vi "Get Source Files And Folders.vi"(8 "Error In":errorcluster, 11 "Configuration":T1) -> (0 "Error Out":errorcluster, 1 "All Source Folders":path[](array[path]), 2 "All Source Files":path[](array[path]), 3 "Configuration":T1)   [LabVIEW 2011, in "LVH-Build-Tools.lvlib"]
uses:
  LVH-Build-Tools.lvlib
  Type Defs/Configuration.ctl
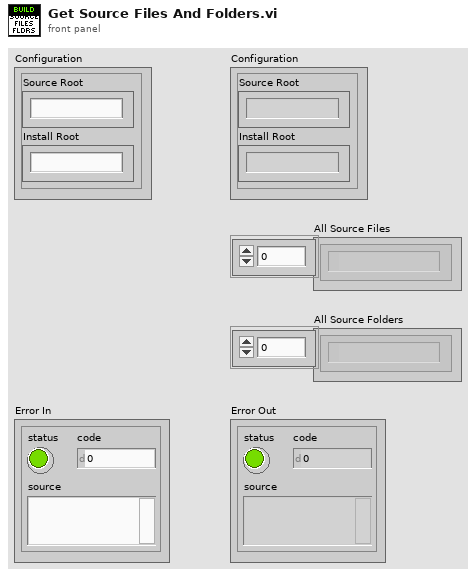
[diagram p1: front panel]
types:
  T1 = typedef "LVH-Build-Tools.lvlib/Configuration.ctl" = cluster{"Source Root":string, "Install Root":string, "Components":string[], "Ignore":string[]}
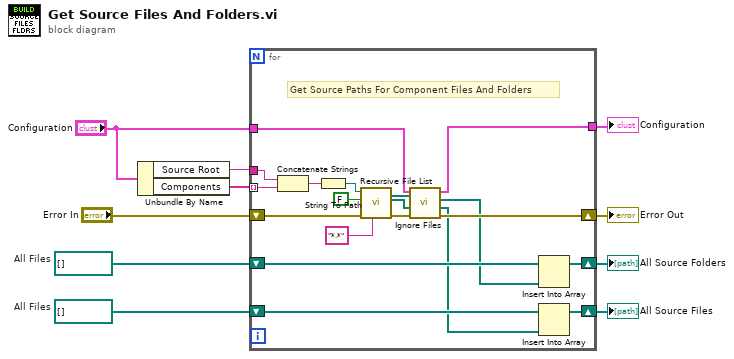
[diagram p0: block diagram]
diagram:
  w7 = path[] []  # All Files
  w6 = path[] []  # All Files
  n1 = Unbundle By Name("Configuration") -> ("Source Root"=w4:string, "Components"=w3:string[])
  n2 = for {
    tunnel: w3 -> [w17] mode=indexing
    tunnel: w4 -> [w18]
    shift-right: [w23] -> w8
    shift-left: w6 -> [w22]
    shift-right: [w20] -> w10
    shift-left: w7 -> [w21]
    shift-right: [w19] -> w9
    shift-left: "Error In" -> [w24]
    tunnel: "Configuration" -> [w14]
    tunnel: [w13] -> w1
    # "Get Source Paths For Component Files And Folders"
    n3 = Concatenate Strings(w18, w17) -> (w25:string)
    n4 = String To Path(string=w25) -> (path=w26:path)
    n5 = call <vilib>:"Recursive File List.vi"("pattern"="*.*", "error in (no error)"=w24, "Treat LLBs as Folders?"=FALSE, "Folder Path"=w26) -> ("error out"=w29:errorcluster, "All Files in Dir"=w15:path[], "All Folders"=w16:path[])  [unwired: 3 in, 2 out]
    n6 = call "Ignore Files.vi"("Error In"=w29, "All Files"=w15, "All Folders"=w16, "Configuration"=w14) -> ("Error Out"=w19:errorcluster, "All Files"=w11:path[], "All Folders"=w12:path[], "Configuration"=w13:T1)  [unwired: 4 in]
    n7 = Insert Into Array(array=w22, new element=w12) -> (w23:path[])  [unwired: 1 in]
    n8 = Insert Into Array(array=w21, new element=w11) -> (w20:path[])  [unwired: 1 in]
  }
  "All Source Files" <- w10
  "Error Out" <- w9
  "All Source Folders" <- w8
  "Configuration" <- w1
